vi "Get Column Data.vi"(8 "error in (no error)":errorcluster, 10 "Header":string, 11 "SLL Spreadsheet in":refnum<class "SLL Table.lvclass">) -> (0 "error out":errorcluster, 1 "Found?":bool, 2 "Data[]":string[](array[string]), 3 "SLL Spreadsheet out":refnum<class "SLL Table.lvclass">)   [LabVIEW 2014, in "SLL Table.lvclass"]
uses:
  SLL Table.lvclass
  SLL Table.lvclass/SLL Table.ctl
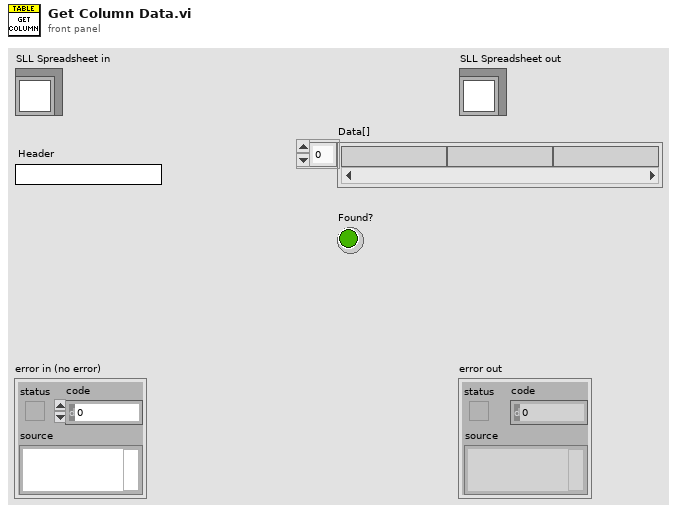
[diagram p1: front panel]
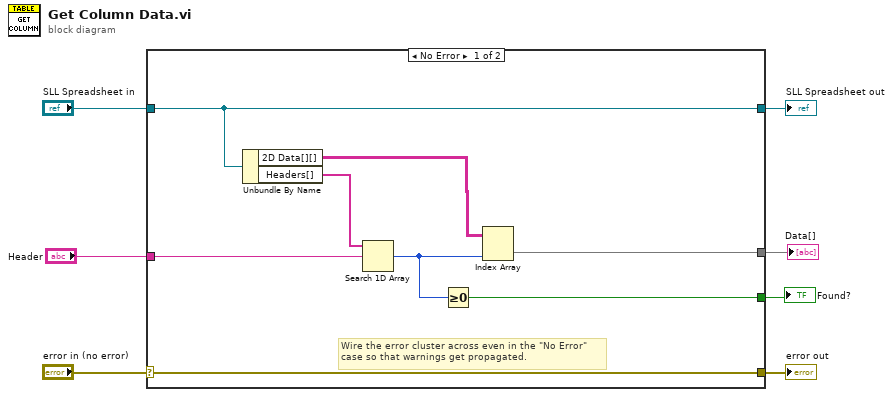
[diagram p0: block diagram]
diagram:
  n1 = case shown="No Error" "error in (no error)" {
    selector: "error in (no error)" -> [w15 w17]
    tunnel: [w15 w17] -> w6
    tunnel: [w14 w16] -> w4
    tunnel: "SLL Spreadsheet in" -> [w14 w16]
    tunnel: "Header" -> [w12 _]
    tunnel: [w11 _] -> w2
    tunnel: [w8 _] -> w1
    frame No Error {
      # "Wire the error cluster across even in the \"No Error\"\ncase so that warnings get propagated."
      n2 = Unbundle By Name(w14) -> ("2D Data[][]"=w10:string[][], "Headers[]"=w13:string[])
      n3 = Search 1D Array(1D array=w13, element=w12) -> (index of element=w9:i32)  [unwired: 1 in]
      n4 = Greater Or Equal To 0?(x=w9) -> (x >= 0?=w8:bool)
      n5 = Index Array(array=w10, index (col)=w9) -> (element=w11:string[])  [unwired: 1 in]
    }
    frame Error {
    }
  }
  "error out" <- w6
  "SLL Spreadsheet out" <- w4
  "Data[]" <- w2
  "Found?" <- w1
